vi "DIO mode set.vi"(8 "error in (no error)":errorcluster, 10 "mode":enum16{"input", "output"}(ring), 11 "DIO in":refnum<class "DIO.lvclass">) -> (0 "error out":errorcluster, 3 "DIO out":refnum<class "DIO.lvclass">)   [LabVIEW 2019, in "my FPGA lib.lvlib" / "DIO.lvclass"]
uses:
  DIO.lvclass
  DIO.lvclass/DIO.ctl
  <vilib>/Utility/error.llb/Error Cluster From Error Code.vi
  <vilib>/rvi/errors/niLvFpgaAdjustHostInterfaceError.vi
  <vilib>/rvi/interface/nirviReadWriteControl/nirviReadWriteControl.xnode
  NiFpgaLv.dll
  <vilib>/rvi/interface/Simulation/niFpgaSimulationCallBeginRW.vi
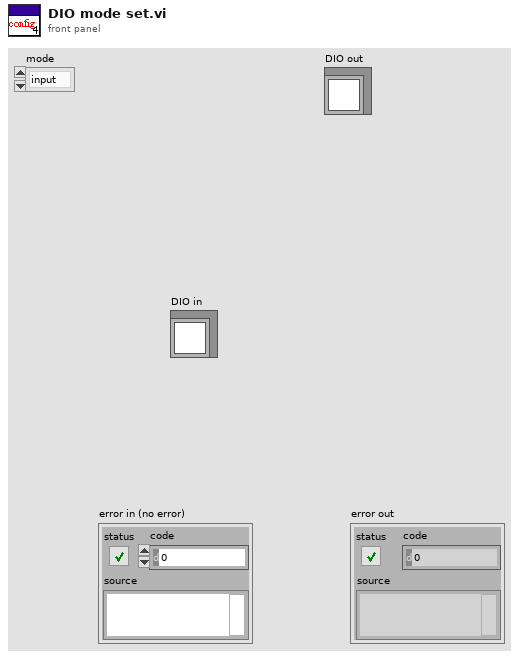
[diagram p1: front panel]
types:
  T1 = typedef "my FPGA lib.lvlib/DIO.lvclass/DIO enum.ctl" = enum16{"US.1", "US.2", "US.3", "US.4", "C.0", "C.1", "C.2", "C.3", "C.4", "C.5", "C.6", "C.7", "B.14", "B.15"}
  T2 = typedef "my FPGA lib.lvlib/DIO.lvclass/port.ctl" = enum16{"US", "C.", "B."}
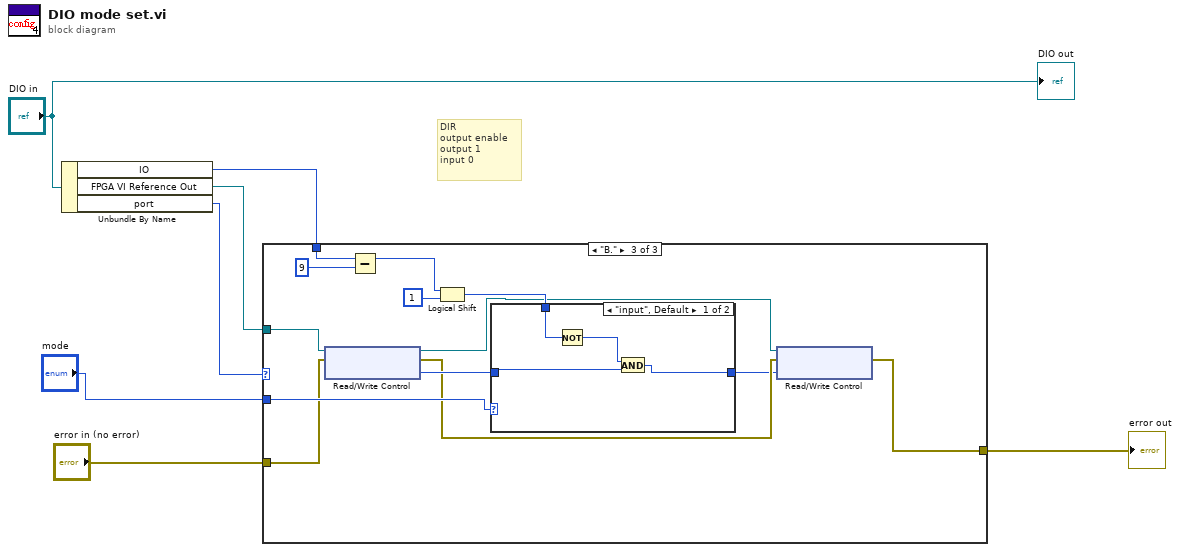
[diagram p0: block diagram]
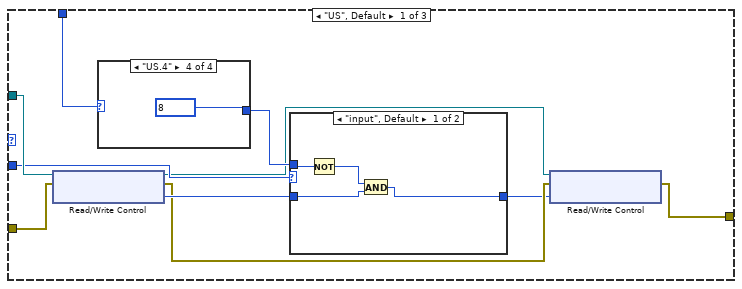
[diagram p2: hidden frame]
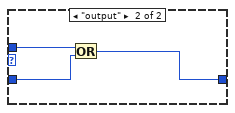
[diagram p3: hidden frame]
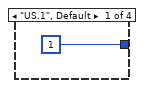
[diagram p4: hidden frame]
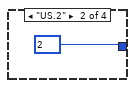
[diagram p5: hidden frame]
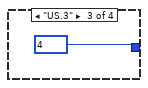
[diagram p6: hidden frame]
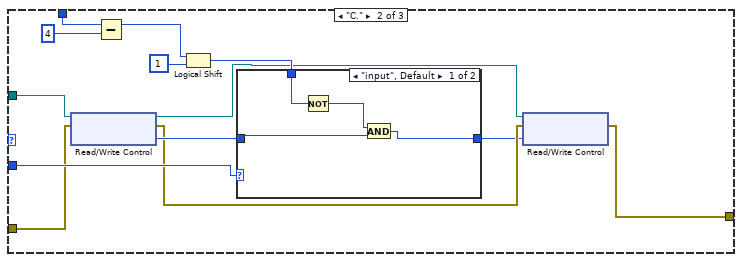
[diagram p7: hidden frame]
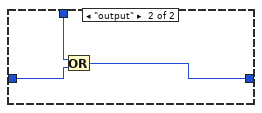
[diagram p8: hidden frame]
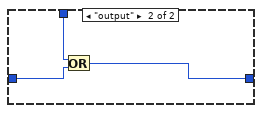
[diagram p9: hidden frame]
diagram:
  # "DIR\noutput enable\noutput 1\ninput 0"
  n1 = Unbundle By Name("DIO in") -> ("IO"=w5:T1, "FPGA VI Reference Out"=w3:refnum<k20>, "port"=w6:T2)
  n2 = case shown="\"B.\"" w6 {
    tunnel: w5 -> [w17 w40 w60]
    tunnel: "error in (no error)" -> [w15 w37 w57]
    tunnel: w3 -> [w16 w38 w58]
    tunnel: "mode" -> [w14 w39 w59]
    tunnel: [w8 w31 w51] -> w1
    frame "US", Default {
      n3 = xnode "Read/Write Control"("FPGA VI Reference In"=w16, "error in"=w15) -> ("FPGA VI Reference Out"=w11:refnum<k20>, "error out"=w10:errorcluster, "Ultrasonic.io.DIR"=w12:u8)
      n4 = case shown="\"US.4\"" w17 {
        tunnel: [u8 1 u8 2 u8 4 u8 8] -> w13
        frame "US.1", Default {
        }
        frame "US.2" {
        }
        frame "US.3" {
        }
        frame "US.4" {
        }
      }
      n5 = case shown="\"input\", Default" w14 {
        tunnel: w13 -> [w21 w24]
        tunnel: w12 -> [w19 w23]
        tunnel: [w18 w22] -> w9
        frame "input", Default {
          n6 = Not(x=w21) -> (.not. x?=w20:u8)
          n7 = And(x=w20, y=w19) -> (x .and. y?=w18:u8)
        }
        frame "output" {
          n8 = Or(x=w24, y=w23) -> (x .or. y?=w22:u8)
        }
      }
      n9 = xnode "Read/Write Control"("FPGA VI Reference In"=w11, "error in"=w10, "Ultrasonic.io.DIR"=w9) -> ("error out"=w8:errorcluster)  [unwired: 1 out]
    }
    frame "C." {
      n10 = xnode "Read/Write Control"("FPGA VI Reference In"=w38, "error in"=w37) -> ("FPGA VI Reference Out"=w34:refnum<k20>, "error out"=w33:errorcluster, "Basic IO DIR"=w35:u8)
      n11 = Subtract(x=w40, y=4) -> (x-y=w30:i32)
      n12 = Logical Shift(y=w30, x=u8 1) -> (x << y=w36:u8)
      n13 = case shown="\"input\", Default" w39 {
        tunnel: w36 -> [w45 w48]
        tunnel: w35 -> [w43 w47]
        tunnel: [w42 w46] -> w32
        frame "input", Default {
          n14 = Not(x=w45) -> (.not. x?=w44:u8)
          n15 = And(x=w44, y=w43) -> (x .and. y?=w42:u8)
        }
        frame "output" {
          n16 = Or(x=w48, y=w47) -> (x .or. y?=w46:u8)
        }
      }
      n17 = xnode "Read/Write Control"("FPGA VI Reference In"=w34, "error in"=w33, "Basic IO DIR"=w32) -> ("error out"=w31:errorcluster)  [unwired: 1 out]
    }
    frame "B." {
      n18 = xnode "Read/Write Control"("FPGA VI Reference In"=w58, "error in"=w57) -> ("FPGA VI Reference Out"=w54:refnum<k20>, "error out"=w53:errorcluster, "Basic.2 IO DIR"=w55:u8)
      n19 = Subtract(x=w60, y=9) -> (x-y=w50:i32)
      n20 = Logical Shift(y=w50, x=u8 1) -> (x << y=w56:u8)
      n21 = case shown="\"input\", Default" w59 {
        tunnel: w56 -> [w65 w68]
        tunnel: w55 -> [w63 w67]
        tunnel: [w62 w66] -> w52
        frame "input", Default {
          n22 = Not(x=w65) -> (.not. x?=w64:u8)
          n23 = And(x=w64, y=w63) -> (x .and. y?=w62:u8)
        }
        frame "output" {
          n24 = Or(x=w68, y=w67) -> (x .or. y?=w66:u8)
        }
      }
      n25 = xnode "Read/Write Control"("FPGA VI Reference In"=w54, "error in"=w53, "Basic.2 IO DIR"=w52) -> ("error out"=w51:errorcluster)  [unwired: 1 out]
    }
  }
  "error out" <- w1
  "DIO out" <- "DIO in"
